vi "HumanButtonBoxReefHeightsInOrOut.vi"(5 "Outtake":bool, 7 "Intake":bool, 8 "Barge/Processor?":bool, 9 "CoralFloor/Source?":bool, 10 "A1/A2/AlgFloor":bool, 11 "L1-L4?":bool) -> (0 "OuttakeAlgae":bool, 1 "IntakeAlgae":bool, 2 "OuttakeCoral":bool, 3 "IntakeCoral":bool)   [LabVIEW 2023]
uses:
  <vilib>/Rock Robotics/WPI/ThirdParty/JAS_Junk/TrajLib/Timer_New.vi
  <vilib>/Utility/semaphor.llb/Obtain Semaphore Reference.vi
  <vilib>/Rock Robotics/WPI/ThirdParty/JAS_Junk/TrajLib/Timer_Reset.vi
  <vilib>/Rock Robotics/WPI/ThirdParty/JAS_Junk/TrajLib/Timer_Start.vi
  <vilib>/Rock Robotics/WPI/ThirdParty/JAS_Junk/TrajLib/Timer_HasPeriodPassedOnce.vi
  <vilib>/Rock Robotics/WPI/ThirdParty/JAS_Junk/TrajLib/Timer_Stop.vi
  <vilib>/Rock Robotics/WPI/ThirdParty/JAS_Junk/TrajLib/Trajectory_Library.lvlib
panel:
  # "elevcoralfloor, source +intake = intake coral\nelevBarge, processor+outtake = outtake algae\nxL1-L4Elev + outtake = outtake coral\nxA1-A2, algFloor + intake = AlgIntake"
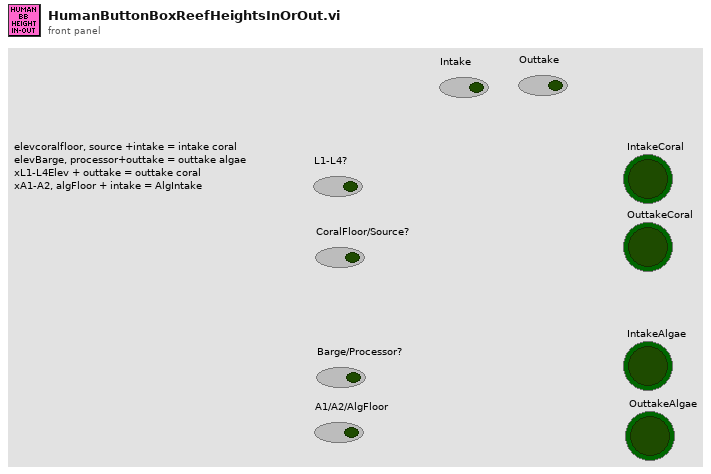
[diagram p1: front panel]
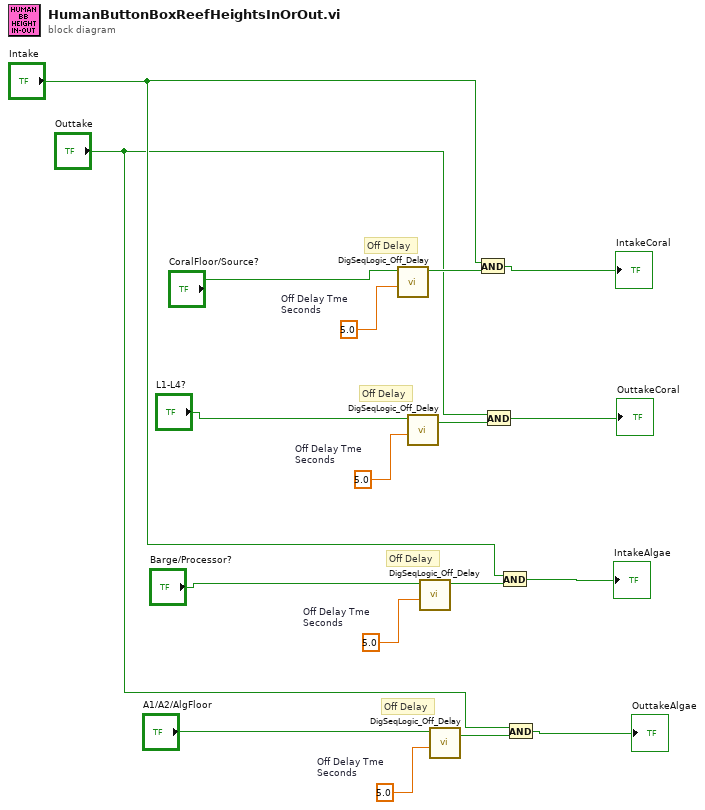
[diagram p0: block diagram]
diagram:
  w8 = 5.0  # Off Delay Tme Seconds
  w10 = 5.0  # Off Delay Tme Seconds
  w16 = 5.0  # Off Delay Tme Seconds
  w18 = 5.0  # Off Delay Tme Seconds
  # "Off Delay"
  # "Off Delay"
  # "Off Delay"
  # "Off Delay"
  n1 = call <vilib>:"DigSeqLogic_Off_Delay.vi"("Delay"=w16, "Input"="CoralFloor/Source?") -> ("Output"=w15:bool)  [unwired: 8 in, 1 out]
  n2 = call <vilib>:"DigSeqLogic_Off_Delay.vi"("Delay"=w18, "Input"="L1-L4?") -> ("Output"=w17:bool)  [unwired: 8 in, 1 out]
  n3 = call <vilib>:"DigSeqLogic_Off_Delay.vi"("Delay"=w8, "Input"="Barge/Processor?") -> ("Output"=w7:bool)  [unwired: 8 in, 1 out]
  n4 = call <vilib>:"DigSeqLogic_Off_Delay.vi"("Delay"=w10, "Input"="A1/A2/AlgFloor") -> ("Output"=w9:bool)  [unwired: 8 in, 1 out]
  n5 = And(x="Intake", y=w15) -> (x .and. y?=→"IntakeCoral":bool)
  n6 = And(x="Outtake", y=w17) -> (x .and. y?=→"OuttakeCoral":bool)
  n7 = And(x="Intake", y=w7) -> (x .and. y?=→"IntakeAlgae":bool)
  n8 = And(x="Outtake", y=w9) -> (x .and. y?=→"OuttakeAlgae":bool)
